vi "DashboardPush.vi"(5 "Joystick 0 Ref":T1, 7 "Joystick 1 Ref":T1) -> ()   [LabVIEW 2018]
uses:
  <vilib>/Rock Robotics/WPI/Joystick/WPI_JoystickDevRef.ctl
  <vilib>/Rock Robotics/WPI/Joystick/WPI_JoystickDeviceEnum.ctl
  1a812ba0-d878-476d-99f2-b93886c55b51.vi
  4ab55bdd-9685-40f0-9085-ecc7bf01abd7.vi
  133b72f1-f6b5-40a0-849f-8c3469abb341.vi
  418ca814-9bf7-4181-a5ae-ea4e15d15a62.vi
  5b9a1c80-d2af-4722-947b-ad6779bb500a.vi
  bbae46cd-89b0-4a78-83b4-a5d1ddadd6d9.vi
  6394f793-1348-457d-85f4-7648f9013d39.vi
  47d326fc-03e5-451f-ae34-c9ea74063880.vi
  a27518ae-5d79-4e43-96da-b3cc959109f2.vi
  a9e42ba8-a108-4121-8da4-7ed463bc445a.vi
  e7382db6-2398-4bf7-9509-2739849d011a.vi
  fb3d1e40-1309-4105-9d60-3501161224b8.vi
  edb44874-fd78-454c-9bff-6d2a69ee6fec.vi
  dfb785ac-7a80-4692-ab1e-e9791fae54f3.vi
  5b13cb5e-6146-47d8-ae09-8b12801406e1.vi
  221b1552-0cc4-4389-bc13-d572fc4176ac.vi
  30f734cc-7591-4d07-939c-c5b43ee5df0c.vi
  d7311573-fb90-4913-8cda-848d1d3ce53b.vi
  7ba6df12-c395-4848-b3a1-04dcd1203c1b.vi
  6301e614-6b7f-47cf-b382-4b27c7e33111.vi
  d83519f1-9582-40c6-a23b-344b6b305b5b.vi
  6aad11fd-ae03-4511-b650-1fa0753debfc.vi
  7035114a-0e6f-4312-ac03-8078da68b1cc.vi
  3bc1cfba-3c18-4848-9658-0328ea52b25d.vi
  ee07aba5-9db9-42ab-a6d0-ff6a71bb383e.vi
  31b97e73-c245-4c28-83b2-b8b7bc5cac65.vi
  8687fe65-8d2d-4f02-ae89-6e8600396bf0.vi
  359c22e3-9c88-41c1-8194-a7f6db251ab3.vi
  9a35cad7-8924-4936-b892-f51ff88f3087.vi
  77a43352-c56d-4a82-a601-0e029bfbecdd.vi
  6c32de76-4603-4c98-9548-18c068db77e4.vi
  fb2c5630-2057-4e14-823f-31378c39dbf8.vi
  d6cbd67f-9b17-42bf-843e-f5ce2d93bab6.vi
  9a319e29-0bce-4b5a-a8ba-81b1ec785933.vi
  c84b3921-0e7b-4db5-8b5b-9ca439e6cec8.vi
  80ca6acc-a426-4631-8635-04e987b8dcbd.vi
  32f607b5-8f1a-4da3-a9f3-63ceddb82894.vi
  SensorReadings.vi
  RobotStates.vi
  Inputs_DriverStation.vi
  <vilib>/Rock Robotics/Network Tables/NT Write Number.vi
  Robot Global Data.vi
  <vilib>/Rock Robotics/Network Tables/NT Write Boolean.vi
panel:
  in  "Level 2 Height":dbl=100.0
  in  "Level 3 Height":dbl=200.0
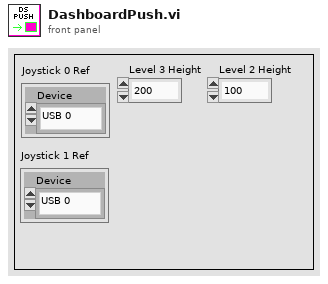
[diagram p1: front panel]
types:
  T1 = typedef "WPI_JoystickDevRef.ctl" = cluster{"Device":T2}
  T2 = typedef "WPI_JoystickDeviceEnum.ctl" = enum16{"USB 0", "USB 1", "USB 2", "USB 3", "USB 4", "USB 5"}
  T3 = cluster{"[0]":bool, "[1]":bool, "[2]":bool, "[3]":bool, "[4]":bool, "[5]":bool, "[6]":bool, "[7]":bool, "[8]":bool, "[9]":bool, "[10]":bool, "[11]":bool, "[12]":bool, "[13]":bool}
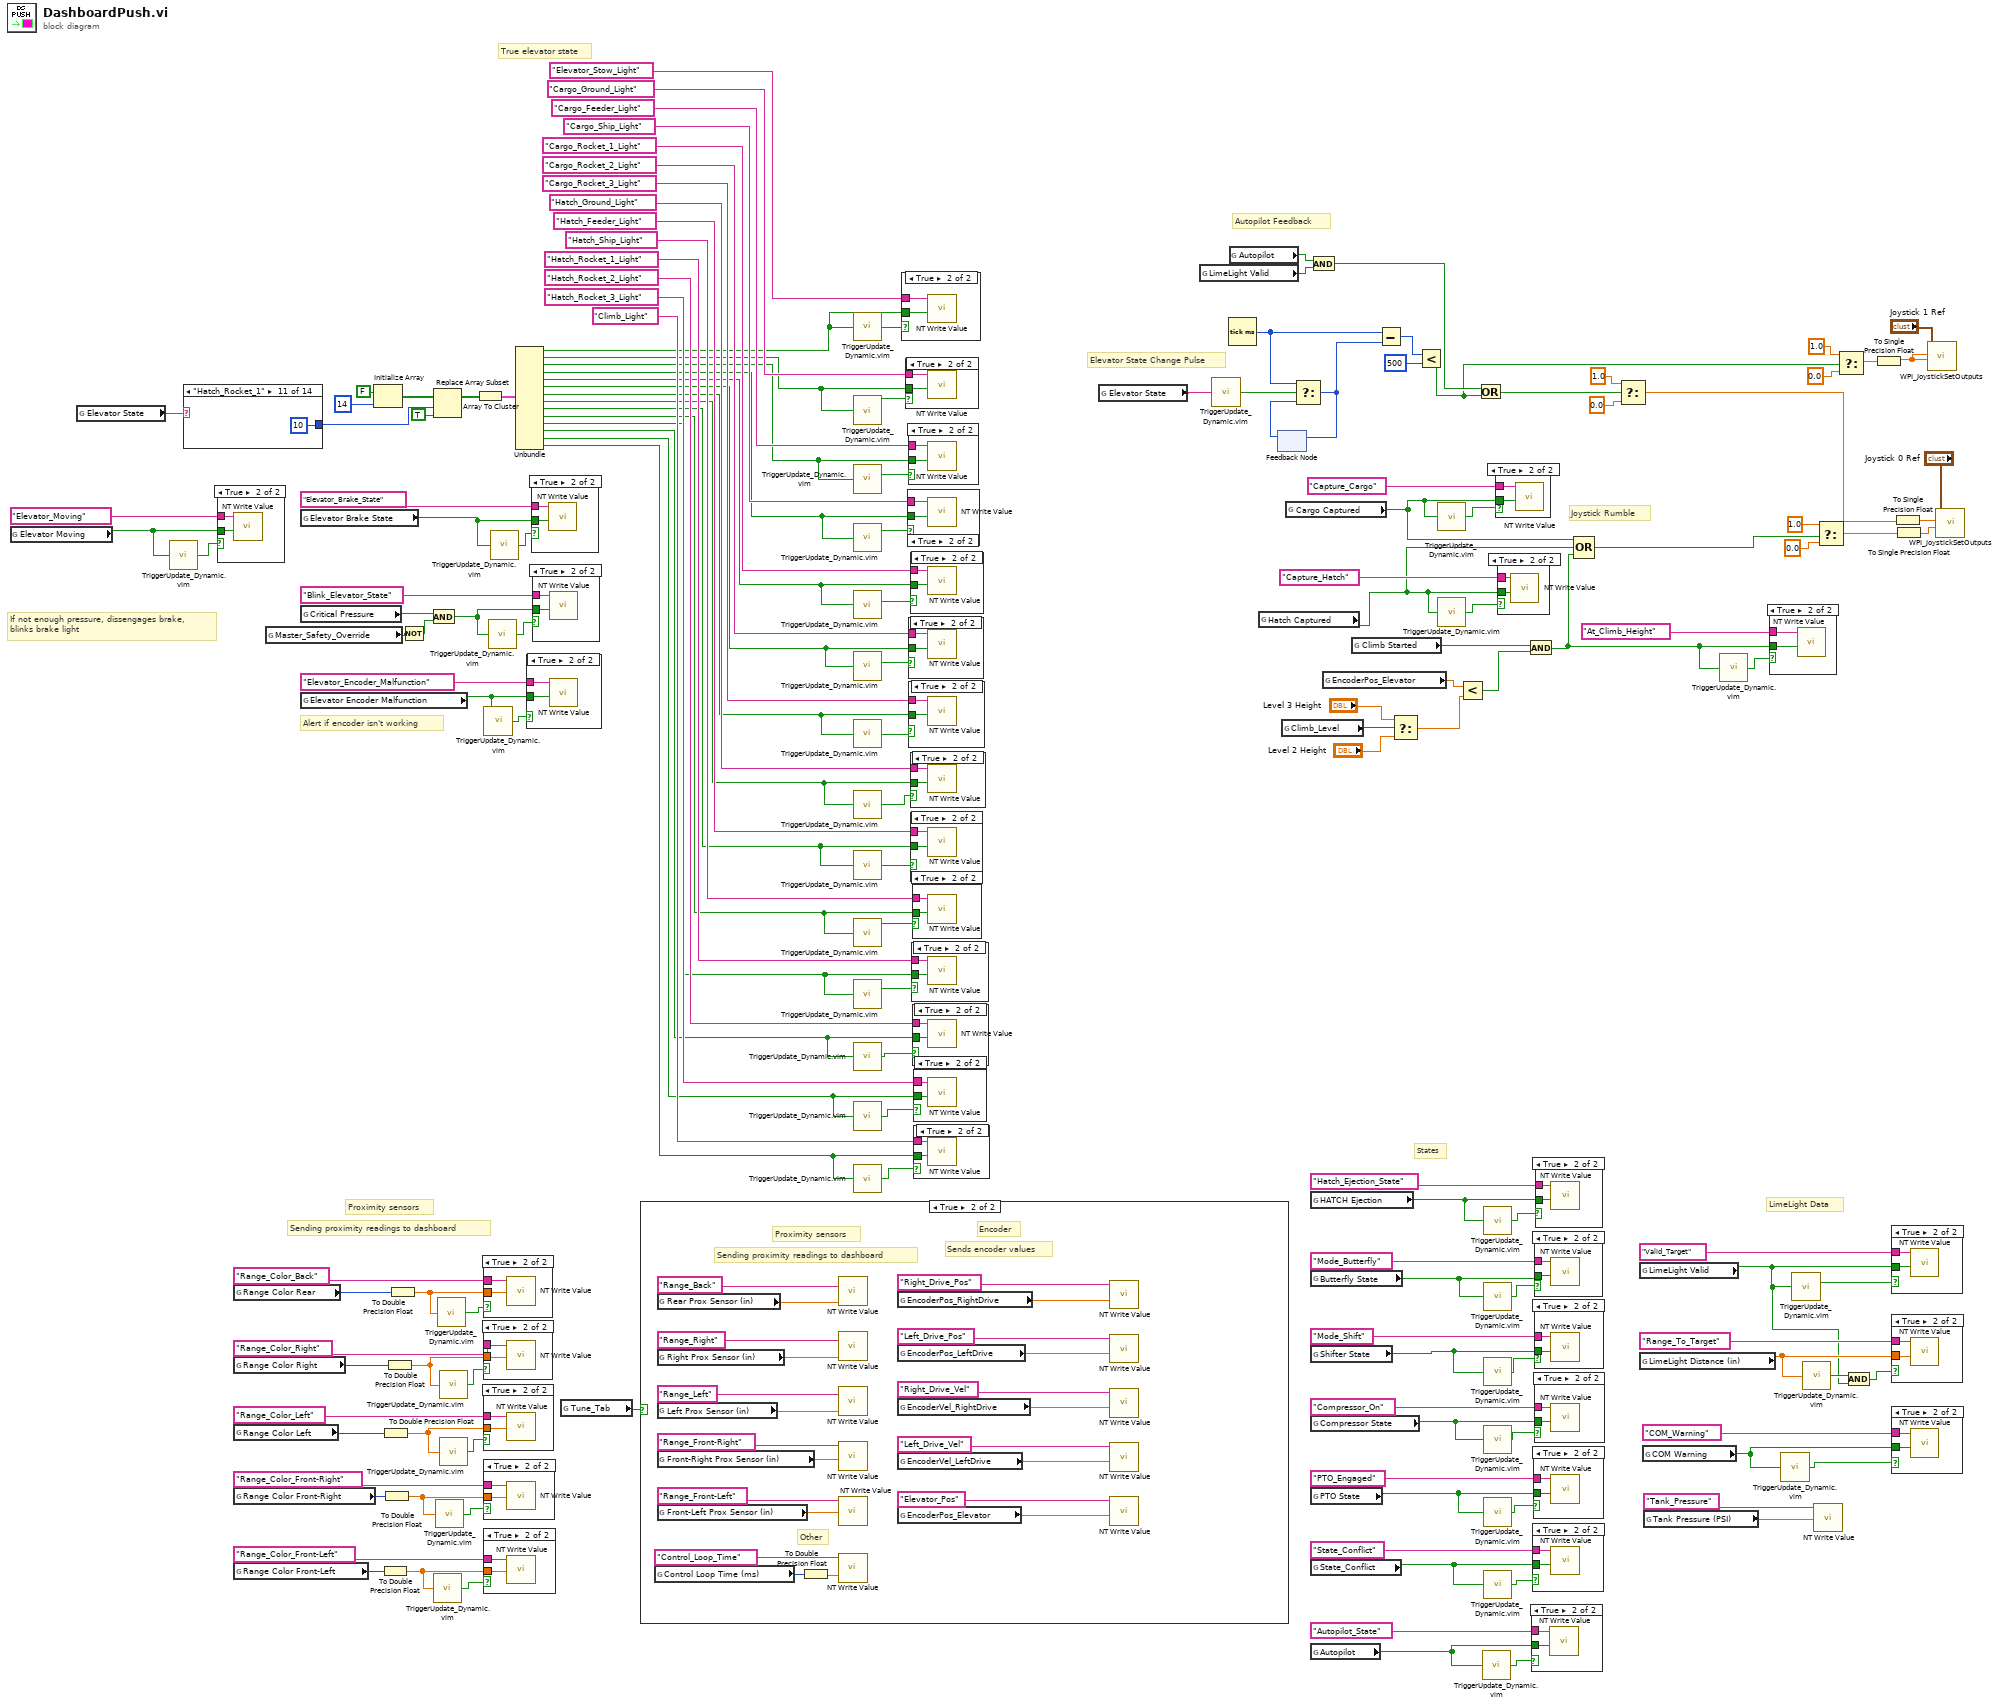
[diagram p0: block diagram]
diagram:
  # "States"
  # "Elevator State Change Pulse"
  # "LimeLight Data"
  # "Autopilot Feedback"
  # "Sending proximity readings to dashboard"
  # "Alert if encoder isn't working"
  # "If not enough pressure, dissengages brake,\nblinks brake light"
  # "Joystick Rumble"
  # "Proximity sensors"
  # "True elevator state"
  n1 = global read "RobotStates.vi" "Elevator Moving"() -> (w6:bool)
  n2 = global read "RobotStates.vi" "Elevator State"() -> (w129:string)
  n3 = call "TriggerUpdate_Dynamic.vim"("Trigger"=w6) -> ("Update"=w5:bool)
  n4 = case shown="\"Hatch_Rocket_1\"" w129 {
    tunnel: [0 1 2 3 4 5 6 7 8 9 10 11 12 13] -> w128
    frame "Elevator_Stow", Default {
    }
    frame "Cargo_Ground" {
    }
    frame "Cargo_Feeder" {
    }
    frame "Cargo_Ship" {
    }
    frame "Cargo_Rocket_1" {
    }
    frame "Cargo_Rocket_2" {
    }
    frame "Cargo_Rocket_3" {
    }
    frame "Hatch_Ground" {
    }
    frame "Hatch_Feeder" {
    }
    frame "Hatch_Ship" {
    }
    frame "Hatch_Rocket_1" {
    }
    frame "Hatch_Rocket_2" {
    }
    frame "Hatch_Rocket_3" {
    }
    frame "Climb" {
    }
  }
  n5 = case shown="True" w5 {
    tunnel: "Elevator_Moving" ("Name") -> [_ w178]
    tunnel: w6 -> [_ w177]
    frame False {
    }
    frame True {
      n6 = call-poly <vilib>:"NT Write Value.vi"("Boolean"=w177, "Name"=w178) -> ()  [unwired: 9 in, 1 out]
    }
  }
  n7 = global read "SensorReadings.vi" "Range Color Rear"() -> (w155:u32)
  n8 = global read "SensorReadings.vi" "Range Color Right"() -> (w153:u32)
  n9 = global read "SensorReadings.vi" "Range Color Left"() -> (w151:u32)
  n10 = global read "SensorReadings.vi" "Range Color Front-Right"() -> (w149:u32)
  n11 = global read "SensorReadings.vi" "Range Color Front-Left"() -> (w124:u32)
  n12 = global read "Inputs_DriverStation.vi" "Master_Safety_Override"() -> (w110:bool)
  n13 = global read "RobotStates.vi" "Elevator Brake State"() -> (w51:bool)
  n14 = global read "SensorReadings.vi" "Critical Pressure"() -> (w111:bool)
  n15 = global read "SensorReadings.vi" "Elevator Encoder Malfunction"() -> (w1:bool)
  n16 = Initialize Array(FALSE, 14 ("dimension size")) -> (w134:bool[])
  n17 = To Double Precision Float(number=w124) -> (double precision float=w55:dbl)
  n18 = To Double Precision Float(number=w151) -> (double precision float=w59:dbl)
  n19 = To Double Precision Float(number=w149) -> (double precision float=w57:dbl)
  n20 = To Double Precision Float(number=w153) -> (double precision float=w61:dbl)
  n21 = To Double Precision Float(number=w155) -> (double precision float=w63:dbl)
  n22 = Not(x=w110) -> (.not. x?=w109:bool)
  n23 = And(x=w111, y=w109) -> (x .and. y?=w47:bool)
  n24 = Replace Array Subset(array=w134, new element=TRUE ("new element/subarray"), index=w128) -> (w132:bool[])
  n25 = call "TriggerUpdate_Dynamic.vim"("Trigger"=w55) -> ("Update"=w54:bool)
  n26 = call "TriggerUpdate_Dynamic.vim"("Trigger"=w57) -> ("Update"=w56:bool)
  n27 = call "TriggerUpdate_Dynamic.vim"("Trigger"=w63) -> ("Update"=w62:bool)
  n28 = call "TriggerUpdate_Dynamic.vim"("Trigger"=w61) -> ("Update"=w60:bool)
  n29 = call "TriggerUpdate_Dynamic.vim"("Trigger"=w59) -> ("Update"=w58:bool)
  n30 = Array To Cluster(array=w132) -> (cluster=w131:T3)
  n31 = case shown="True" w60 {
    tunnel: "Range_Color_Right" ("refnum name") -> [_ w180]
    tunnel: w61 -> [_ w179]
    frame False {
    }
    frame True {
      n32 = call-poly <vilib>:"NT Write Value.vi"("Numeric"=w179, "Name"=w180) -> ()  [unwired: 9 in, 1 out]
    }
  }
  n33 = case shown="True" w58 {
    tunnel: "Range_Color_Left" ("refnum name") -> [_ w182]
    tunnel: w59 -> [_ w181]
    frame False {
    }
    frame True {
      n34 = call-poly <vilib>:"NT Write Value.vi"("Numeric"=w181, "Name"=w182) -> ()  [unwired: 9 in, 1 out]
    }
  }
  n35 = call "TriggerUpdate_Dynamic.vim"("Trigger"=w1) -> ("Update"=w52:bool)
  n36 = case shown="True" w62 {
    tunnel: "Range_Color_Back" ("refnum name") -> [_ w184]
    tunnel: w63 -> [_ w183]
    frame False {
    }
    frame True {
      n37 = call-poly <vilib>:"NT Write Value.vi"("Numeric"=w183, "Name"=w184) -> ()  [unwired: 9 in, 1 out]
    }
  }
  n38 = case shown="True" w56 {
    tunnel: "Range_Color_Front-Right" ("refnum name") -> [_ w186]
    tunnel: w57 -> [_ w185]
    frame False {
    }
    frame True {
      n39 = call-poly <vilib>:"NT Write Value.vi"("Numeric"=w185, "Name"=w186) -> ()  [unwired: 9 in, 1 out]
    }
  }
  n40 = case shown="True" w54 {
    tunnel: w55 -> [_ w188]
    tunnel: "Range_Color_Front-Left" ("refnum name") -> [_ w187]
    frame False {
    }
    frame True {
      n41 = call-poly <vilib>:"NT Write Value.vi"("Numeric"=w188, "Name"=w187) -> ()  [unwired: 9 in, 1 out]
    }
  }
  n42 = call "TriggerUpdate_Dynamic.vim"("Trigger"=w47) -> ("Update"=w49:bool)
  n43 = call "TriggerUpdate_Dynamic.vim"("Trigger"=w51) -> ("Update"=w50:bool)
  n44 = Unbundle(w131) -> ("[0]"=w108:bool, "[1]"=w106:bool, "[2]"=w104:bool, "[3]"=w102:bool, "[4]"=w100:bool, "[5]"=w98:bool, "[6]"=w96:bool, "[7]"=w94:bool, "[8]"=w92:bool, "[9]"=w90:bool, "[10]"=w88:bool, "[11]"=w86:bool, "[12]"=w84:bool, "[13]"=w82:bool)
  n45 = case shown="True" w52 {
    tunnel: "Elevator_Encoder_Malfunction" ("Name") -> [_ w190]
    tunnel: w1 -> [_ w189]
    frame False {
    }
    frame True {
      n46 = call-poly <vilib>:"NT Write Value.vi"("Boolean"=w189, "Name"=w190) -> ()  [unwired: 9 in, 1 out]
    }
  }
  n47 = case shown="True" w50 {
    tunnel: "Elevator_Brake_State" ("Name") -> [_ w192]
    tunnel: w51 -> [_ w191]
    frame False {
    }
    frame True {
      n48 = call-poly <vilib>:"NT Write Value.vi"("Boolean"=w191, "Name"=w192) -> ()  [unwired: 9 in, 1 out]
    }
  }
  n49 = case shown="True" w49 {
    tunnel: "Blink_Elevator_State" ("Name") -> [_ w194]
    tunnel: w47 -> [_ w193]
    frame False {
    }
    frame True {
      n50 = call-poly <vilib>:"NT Write Value.vi"("Boolean"=w193, "Name"=w194) -> ()  [unwired: 9 in, 1 out]
    }
  }
  n51 = global read "Inputs_DriverStation.vi" "Tune_Tab"() -> (w53:bool)
  n52 = case shown="True" w53 {
    frame False {
    }
    frame True {
      # "Sending proximity readings to dashboard"
      # "Proximity sensors"
      # "Sends encoder values"
      # "Other"
      # "Encoder"
      n53 = global read "SensorReadings.vi" "Control Loop Time (ms)"() -> (w196:u32)
      n54 = global read "SensorReadings.vi" "Rear Prox Sensor (in)"() -> (w216:dbl)
      n55 = global read "SensorReadings.vi" "Right Prox Sensor (in)"() -> (w214:dbl)
      n56 = global read "SensorReadings.vi" "Left Prox Sensor (in)"() -> (w212:dbl)
      n57 = global read "SensorReadings.vi" "Front-Right Prox Sensor (in)"() -> (w210:dbl)
      n58 = global read "SensorReadings.vi" "Front-Left Prox Sensor (in)"() -> (w198:dbl)
      n59 = To Double Precision Float(number=w196) -> (double precision float=w195:dbl)
      n60 = call-poly <vilib>:"NT Write Value.vi"("Numeric"=w216, "Name"="Range_Back") -> ()  [unwired: 9 in, 1 out]
      n61 = call-poly <vilib>:"NT Write Value.vi"("Numeric"=w214, "Name"="Range_Right") -> ()  [unwired: 9 in, 1 out]
      n62 = call-poly <vilib>:"NT Write Value.vi"("Numeric"=w212, "Name"="Range_Left") -> ()  [unwired: 9 in, 1 out]
      n63 = call-poly <vilib>:"NT Write Value.vi"("Numeric"=w210, "Name"="Range_Front-Right") -> ()  [unwired: 9 in, 1 out]
      n64 = call-poly <vilib>:"NT Write Value.vi"("Numeric"=w198, "Name"="Range_Front-Left") -> ()  [unwired: 9 in, 1 out]
      n65 = call-poly <vilib>:"NT Write Value.vi"("Numeric"=w195, "Name"="Control_Loop_Time") -> ()  [unwired: 9 in, 1 out]
      n66 = global read "SensorReadings.vi" "EncoderPos_RightDrive"() -> (w209:dbl)
      n67 = global read "SensorReadings.vi" "EncoderPos_LeftDrive"() -> (w207:dbl)
      n68 = global read "SensorReadings.vi" "EncoderVel_RightDrive"() -> (w205:dbl)
      n69 = global read "SensorReadings.vi" "EncoderVel_LeftDrive"() -> (w203:dbl)
      n70 = global read "SensorReadings.vi" "EncoderPos_Elevator"() -> (w201:dbl)
      n71 = call-poly <vilib>:"NT Write Value.vi"("Numeric"=w209, "Name"="Right_Drive_Pos") -> ()  [unwired: 9 in, 1 out]
      n72 = call-poly <vilib>:"NT Write Value.vi"("Numeric"=w207, "Name"="Left_Drive_Pos") -> ()  [unwired: 9 in, 1 out]
      n73 = call-poly <vilib>:"NT Write Value.vi"("Numeric"=w205, "Name"="Right_Drive_Vel") -> ()  [unwired: 9 in, 1 out]
      n74 = call-poly <vilib>:"NT Write Value.vi"("Numeric"=w203, "Name"="Left_Drive_Vel") -> ()  [unwired: 9 in, 1 out]
      n75 = call-poly <vilib>:"NT Write Value.vi"("Numeric"=w201, "Name"="Elevator_Pos") -> ()  [unwired: 9 in, 1 out]
    }
  }
  n76 = call "TriggerUpdate_Dynamic.vim"("Trigger"=w108) -> ("Update"=w107:bool)
  n77 = call "TriggerUpdate_Dynamic.vim"("Trigger"=w106) -> ("Update"=w105:bool)
  n78 = call "TriggerUpdate_Dynamic.vim"("Trigger"=w104) -> ("Update"=w103:bool)
  n79 = call "TriggerUpdate_Dynamic.vim"("Trigger"=w102) -> ("Update"=w101:bool)
  n80 = call "TriggerUpdate_Dynamic.vim"("Trigger"=w100) -> ("Update"=w99:bool)
  n81 = call "TriggerUpdate_Dynamic.vim"("Trigger"=w98) -> ("Update"=w97:bool)
  n82 = call "TriggerUpdate_Dynamic.vim"("Trigger"=w96) -> ("Update"=w95:bool)
  n83 = call "TriggerUpdate_Dynamic.vim"("Trigger"=w94) -> ("Update"=w93:bool)
  n84 = call "TriggerUpdate_Dynamic.vim"("Trigger"=w92) -> ("Update"=w91:bool)
  n85 = call "TriggerUpdate_Dynamic.vim"("Trigger"=w90) -> ("Update"=w89:bool)
  n86 = call "TriggerUpdate_Dynamic.vim"("Trigger"=w88) -> ("Update"=w87:bool)
  n87 = call "TriggerUpdate_Dynamic.vim"("Trigger"=w86) -> ("Update"=w85:bool)
  n88 = call "TriggerUpdate_Dynamic.vim"("Trigger"=w84) -> ("Update"=w83:bool)
  n89 = call "TriggerUpdate_Dynamic.vim"("Trigger"=w82) -> ("Update"=w81:bool)
  n90 = case shown="True" w107 {
    tunnel: "Elevator_Stow_Light" ("refnum name") -> [_ w219]
    tunnel: w108 -> [_ w218]
    frame False {
    }
    frame True {
      n91 = call-poly <vilib>:"NT Write Value.vi"("Boolean"=w218, "Name"=w219) -> ()  [unwired: 9 in, 1 out]
    }
  }
  n92 = case shown="True" w105 {
    tunnel: "Cargo_Ground_Light" ("refnum name") -> [_ w221]
    tunnel: w106 -> [_ w220]
    frame False {
    }
    frame True {
      n93 = call-poly <vilib>:"NT Write Value.vi"("Boolean"=w220, "Name"=w221) -> ()  [unwired: 9 in, 1 out]
    }
  }
  n94 = case shown="True" w101 {
    tunnel: "Cargo_Ship_Light" ("refnum name") -> [_ w223]
    tunnel: w102 -> [_ w222]
    frame False {
    }
    frame True {
      n95 = call-poly <vilib>:"NT Write Value.vi"("Boolean"=w222, "Name"=w223) -> ()  [unwired: 9 in, 1 out]
    }
  }
  n96 = case shown="True" w103 {
    tunnel: "Cargo_Feeder_Light" ("refnum name") -> [_ w225]
    tunnel: w104 -> [_ w224]
    frame False {
    }
    frame True {
      n97 = call-poly <vilib>:"NT Write Value.vi"("Boolean"=w224, "Name"=w225) -> ()  [unwired: 9 in, 1 out]
    }
  }
  n98 = case shown="True" w97 {
    tunnel: "Cargo_Rocket_2_Light" ("refnum name") -> [_ w227]
    tunnel: w98 -> [_ w226]
    frame False {
    }
    frame True {
      n99 = call-poly <vilib>:"NT Write Value.vi"("Boolean"=w226, "Name"=w227) -> ()  [unwired: 9 in, 1 out]
    }
  }
  n100 = case shown="True" w95 {
    tunnel: "Cargo_Rocket_3_Light" ("refnum name") -> [_ w229]
    tunnel: w96 -> [_ w228]
    frame False {
    }
    frame True {
      n101 = call-poly <vilib>:"NT Write Value.vi"("Boolean"=w228, "Name"=w229) -> ()  [unwired: 9 in, 1 out]
    }
  }
  n102 = case shown="True" w99 {
    tunnel: "Cargo_Rocket_1_Light" ("refnum name") -> [_ w231]
    tunnel: w100 -> [_ w230]
    frame False {
    }
    frame True {
      n103 = call-poly <vilib>:"NT Write Value.vi"("Boolean"=w230, "Name"=w231) -> ()  [unwired: 9 in, 1 out]
    }
  }
  n104 = case shown="True" w93 {
    tunnel: "Hatch_Ground_Light" ("refnum name") -> [_ w233]
    tunnel: w94 -> [_ w232]
    frame False {
    }
    frame True {
      n105 = call-poly <vilib>:"NT Write Value.vi"("Boolean"=w232, "Name"=w233) -> ()  [unwired: 9 in, 1 out]
    }
  }
  n106 = case shown="True" w91 {
    tunnel: "Hatch_Feeder_Light" ("refnum name") -> [_ w235]
    tunnel: w92 -> [_ w234]
    frame False {
    }
    frame True {
      n107 = call-poly <vilib>:"NT Write Value.vi"("Boolean"=w234, "Name"=w235) -> ()  [unwired: 9 in, 1 out]
    }
  }
  n108 = case shown="True" w87 {
    tunnel: "Hatch_Rocket_1_Light" ("refnum name") -> [_ w237]
    tunnel: w88 -> [_ w236]
    frame False {
    }
    frame True {
      n109 = call-poly <vilib>:"NT Write Value.vi"("Boolean"=w236, "Name"=w237) -> ()  [unwired: 9 in, 1 out]
    }
  }
  n110 = case shown="True" w89 {
    tunnel: "Hatch_Ship_Light" ("refnum name") -> [_ w239]
    tunnel: w90 -> [_ w238]
    frame False {
    }
    frame True {
      n111 = call-poly <vilib>:"NT Write Value.vi"("Boolean"=w238, "Name"=w239) -> ()  [unwired: 9 in, 1 out]
    }
  }
  n112 = case shown="True" w85 {
    tunnel: "Hatch_Rocket_2_Light" ("refnum name") -> [_ w241]
    tunnel: w86 -> [_ w240]
    frame False {
    }
    frame True {
      n113 = call-poly <vilib>:"NT Write Value.vi"("Boolean"=w240, "Name"=w241) -> ()  [unwired: 9 in, 1 out]
    }
  }
  n114 = case shown="True" w83 {
    tunnel: "Hatch_Rocket_3_Light" ("refnum name") -> [_ w243]
    tunnel: w84 -> [_ w242]
    frame False {
    }
    frame True {
      n115 = call-poly <vilib>:"NT Write Value.vi"("Boolean"=w242, "Name"=w243) -> ()  [unwired: 9 in, 1 out]
    }
  }
  n116 = case shown="True" w81 {
    tunnel: "Climb_Light" ("refnum name") -> [_ w245]
    tunnel: w82 -> [_ w244]
    frame False {
    }
    frame True {
      n117 = call-poly <vilib>:"NT Write Value.vi"("Boolean"=w244, "Name"=w245) -> ()  [unwired: 9 in, 1 out]
    }
  }
  n118 = global read "RobotStates.vi" "Elevator State"() -> (w22:string)
  n119 = global read "SensorReadings.vi" "LimeLight Valid"() -> (w45:bool)
  n120 = call "TriggerUpdate_Dynamic.vim"("Trigger"=w22) -> ("Update"=w14:bool)
  n121 = Tick Count (ms)() -> (millisecond timer value=w18:u32)
  n122 = global read "RobotStates.vi" "Autopilot"() -> (w46:bool)
  n123 = global read "SensorReadings.vi" "Hatch Captured"() -> (w23:bool)
  n124 = feedback #1() -> (w19:u32)  [unwired: 1 in]
  n125 = global read "Inputs_DriverStation.vi" "Climb_Level"() -> (w118:bool)
  n126 = global read "SensorReadings.vi" "Cargo Captured"() -> (w77:bool)
  n127 = Select(t=w18, s=w14, f=w19) -> (s? t:f=w17:u32)
  n128 = feedback-in #1(w17) -> ()
  n129 = And(x=w46, y=w45) -> (x .and. y?=w21:bool)
  n130 = global read "RobotStates.vi" "HATCH Ejection"() -> (w75:bool)
  n131 = global read "RobotStates.vi" "Butterfly State"() -> (w73:bool)
  n132 = global read "RobotStates.vi" "Shifter State"() -> (w71:bool)
  n133 = global read "RobotStates.vi" "Compressor State"() -> (w69:bool)
  n134 = global read "RobotStates.vi" "PTO State"() -> (w67:bool)
  n135 = global read "RobotStates.vi" "State_Conflict"() -> (w65:bool)
  n136 = global read "RobotStates.vi" "Autopilot"() -> (w34:bool)
  n137 = global read "SensorReadings.vi" "EncoderPos_Elevator"() -> (w119:dbl)
  n138 = global read "RobotStates.vi" "Climb Started"() -> (w112:bool)
  n139 = Subtract(x=w18, y=w17) -> (x-y=w16:u32)
  n140 = Select(t="Level 3 Height", s=w118, f="Level 2 Height") -> (s? t:f=w115:dbl)
  n141 = Less?(x=w16, y=u32 500) -> (x < y?=w10:bool)
  n142 = call "TriggerUpdate_Dynamic.vim"("Trigger"=w77) -> ("Update"=w76:bool)
  n143 = call "TriggerUpdate_Dynamic.vim"("Trigger"=w23) -> ("Update"=w78:bool)
  n144 = Less?(x=w119, y=w115) -> (x < y?=w114:bool)
  n145 = Or(x=w21, y=w10) -> (x .or. y?=w20:bool)
  n146 = call "TriggerUpdate_Dynamic.vim"("Trigger"=w34) -> ("Update"=w33:bool)
  n147 = call "TriggerUpdate_Dynamic.vim"("Trigger"=w75) -> ("Update"=w74:bool)
  n148 = call "TriggerUpdate_Dynamic.vim"("Trigger"=w73) -> ("Update"=w72:bool)
  n149 = call "TriggerUpdate_Dynamic.vim"("Trigger"=w71) -> ("Update"=w70:bool)
  n150 = call "TriggerUpdate_Dynamic.vim"("Trigger"=w69) -> ("Update"=w68:bool)
  n151 = call "TriggerUpdate_Dynamic.vim"("Trigger"=w67) -> ("Update"=w66:bool)
  n152 = call "TriggerUpdate_Dynamic.vim"("Trigger"=w65) -> ("Update"=w64:bool)
  n153 = case shown="True" w76 {
    tunnel: "Capture_Cargo" ("Name") -> [_ w247]
    tunnel: w77 -> [_ w246]
    frame False {
    }
    frame True {
      n154 = call-poly <vilib>:"NT Write Value.vi"("Boolean"=w246, "Name"=w247) -> ()  [unwired: 9 in, 1 out]
    }
  }
  n155 = case shown="True" w78 {
    tunnel: "Capture_Hatch" ("Name") -> [_ w249]
    tunnel: w23 -> [_ w248]
    frame False {
    }
    frame True {
      n156 = call-poly <vilib>:"NT Write Value.vi"("Boolean"=w248, "Name"=w249) -> ()  [unwired: 9 in, 1 out]
    }
  }
  n157 = And(x=w112, y=w114) -> (x .and. y?=w80:bool)
  n158 = case shown="True" w33 {
    tunnel: w34 -> [_ w251]
    tunnel: "Autopilot_State" ("Name") -> [_ w250]
    frame False {
    }
    frame True {
      n159 = call-poly <vilib>:"NT Write Value.vi"("Boolean"=w251, "Name"=w250) -> ()  [unwired: 9 in, 1 out]
    }
  }
  n160 = case shown="True" w64 {
    tunnel: w65 -> [_ w253]
    tunnel: "State_Conflict" ("Name") -> [_ w252]
    frame False {
    }
    frame True {
      n161 = call-poly <vilib>:"NT Write Value.vi"("Boolean"=w253, "Name"=w252) -> ()  [unwired: 9 in, 1 out]
    }
  }
  n162 = case shown="True" w66 {
    tunnel: "PTO_Engaged" ("Name") -> [_ w255]
    tunnel: w67 -> [_ w254]
    frame False {
    }
    frame True {
      n163 = call-poly <vilib>:"NT Write Value.vi"("Boolean"=w254, "Name"=w255) -> ()  [unwired: 9 in, 1 out]
    }
  }
  n164 = case shown="True" w72 {
    tunnel: "Mode_Butterfly" ("Name") -> [_ w257]
    tunnel: w73 -> [_ w256]
    frame False {
    }
    frame True {
      n165 = call-poly <vilib>:"NT Write Value.vi"("Boolean"=w256, "Name"=w257) -> ()  [unwired: 9 in, 1 out]
    }
  }
  n166 = case shown="True" w70 {
    tunnel: "Mode_Shift" ("Name") -> [_ w259]
    tunnel: w71 -> [_ w258]
    frame False {
    }
    frame True {
      n167 = call-poly <vilib>:"NT Write Value.vi"("Boolean"=w258, "Name"=w259) -> ()  [unwired: 9 in, 1 out]
    }
  }
  n168 = case shown="True" w68 {
    tunnel: "Compressor_On" ("Name") -> [_ w261]
    tunnel: w69 -> [_ w260]
    frame False {
    }
    frame True {
      n169 = call-poly <vilib>:"NT Write Value.vi"("Boolean"=w260, "Name"=w261) -> ()  [unwired: 9 in, 1 out]
    }
  }
  n170 = case shown="True" w74 {
    tunnel: "Hatch_Ejection_State" ("Name") -> [_ w263]
    tunnel: w75 -> [_ w262]
    frame False {
    }
    frame True {
      n171 = call-poly <vilib>:"NT Write Value.vi"("Boolean"=w262, "Name"=w263) -> ()  [unwired: 9 in, 1 out]
    }
  }
  n172 = Compound Arithmetic op=OR(w77, w23, w80) -> (w36:bool)
  n173 = Select(t=1.0, s=w20, f=0.0) -> (s? t:f=w38:dbl)
  n174 = global read "SensorReadings.vi" "LimeLight Valid"() -> (w26:bool)
  n175 = global read "SensorReadings.vi" "LimeLight Distance (in)"() -> (w29:dbl)
  n176 = global read "RobotStates.vi" "COM Warning"() -> (w3:bool)
  n177 = global read "SensorReadings.vi" "Tank Pressure (PSI)"() -> (w25:dbl)
  n178 = call "TriggerUpdate_Dynamic.vim"("Trigger"=w80) -> ("Update"=w79:bool)
  n179 = case shown="True" w79 {
    tunnel: "At_Climb_Height" ("Name") -> [_ w265]
    tunnel: w80 -> [_ w264]
    frame False {
    }
    frame True {
      n180 = call-poly <vilib>:"NT Write Value.vi"("Boolean"=w264, "Name"=w265) -> ()  [unwired: 9 in, 1 out]
    }
  }
  n181 = call "TriggerUpdate_Dynamic.vim"("Trigger"=w3) -> ("Update"=w2:bool)
  n182 = call "TriggerUpdate_Dynamic.vim"("Trigger"=w26) -> ("Update"=w31:bool)
  n183 = call "TriggerUpdate_Dynamic.vim"("Trigger"=w29) -> ("Update"=w28:bool)
  n184 = call-poly <vilib>:"NT Write Value.vi"("Numeric"=w25, "Name"="Tank_Pressure") -> ()  [unwired: 9 in, 1 out]
  n185 = Select(t=1.0, s=w36, f=0.0) -> (s? t:f=w37:dbl)
  n186 = Select(t=1.0, s=w10, f=0.0) -> (s? t:f=w11:dbl)
  n187 = And(x=w28, y=w26) -> (x .and. y?=w27:bool)
  n188 = To Single Precision Float(number=w11) -> (single precision float=w8:sgl)
  n189 = case shown="True" w31 {
    tunnel: w26 -> [_ w267]
    tunnel: "Valid_Target" ("Name") -> [_ w266]
    frame False {
    }
    frame True {
      n190 = call-poly <vilib>:"NT Write Value.vi"("Boolean"=w267, "Name"=w266) -> ()  [unwired: 9 in, 1 out]
    }
  }
  n191 = case shown="True" w27 {
    tunnel: w29 -> [_ w269]
    tunnel: "Range_To_Target" ("Name") -> [_ w268]
    frame False {
    }
    frame True {
      n192 = call-poly <vilib>:"NT Write Value.vi"("Numeric"=w269, "Name"=w268) -> ()  [unwired: 9 in, 1 out]
    }
  }
  n193 = case shown="True" w2 {
    tunnel: w3 -> [_ w271]
    tunnel: "COM_Warning" ("Name") -> [_ w270]
    frame False {
    }
    frame True {
      n194 = call-poly <vilib>:"NT Write Value.vi"("Boolean"=w271, "Name"=w270) -> ()  [unwired: 9 in, 1 out]
    }
  }
  n195 = To Single Precision Float(number=w38) -> (single precision float=w42:sgl)
  n196 = To Single Precision Float(number=w37) -> (single precision float=w39:sgl)
  n197 = call <vilib>:"WPI_JoystickSetOutputs.vi"("Right Rumble"=w8, "Left Rumble"=w8, "JoystickDevRef"="Joystick 1 Ref") -> ()  [unwired: 7 in, 2 out]
  n198 = call <vilib>:"WPI_JoystickSetOutputs.vi"("Right Rumble"=w39, "Left Rumble"=w42, "JoystickDevRef"="Joystick 0 Ref") -> ()  [unwired: 7 in, 2 out]
